vi "Run Tests.vi"(8 "error in (no error)":errorcluster, 10 "Filter":T1, 11 "Execution UI in":refnum<class "Execution UI.lvclass">) -> (0 "error out":errorcluster, 3 "Execution UI out":refnum<class "Execution UI.lvclass">)   [LabVIEW 2020, in "Execution UI.lvclass"]
uses:
  Execution UI.lvclass
  Execution UI.lvclass/Execution UI.ctl
  Process/Process.lvclass
  Result Model by Reference/Result Model by Reference.lvclass
  C:/git/astemes-lunit/source/User Interface/Process/Process.lvclass
  C:/git/astemes-lunit/source/User Interface/Execution UI/Execution UI.lvclass
  C:/git/astemes-lunit/source/Framework/Result Observer/Result Observer.lvclass
  Result Model/Tree Item Filter.ctl
  Result Model/Result Model.lvclass
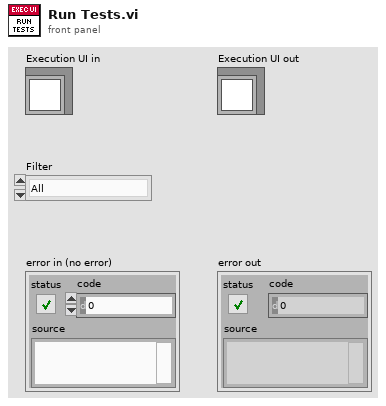
[diagram p1: front panel]
types:
  T1 = typedef "Result Model.lvclass/Tree Item Filter.ctl" = enum16{"All", "Only Fails", "Fails and Not Executed"}
  T2 = cluster{"Left Cell String":string, "Child Text":string[], "Child Tag":string, "Item Indent":i32, "Child Only?":bool, "Glyph Index":i32}[]
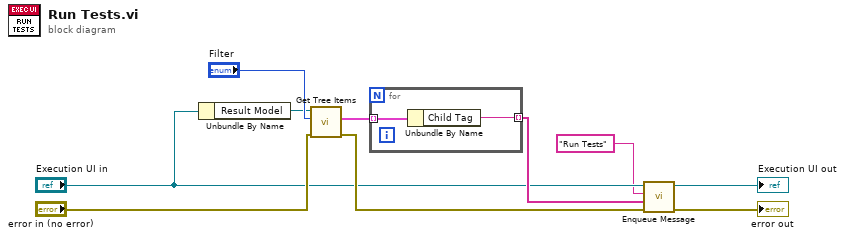
[diagram p0: block diagram]
diagram:
  n1 = Unbundle By Name("Execution UI in") -> ("Result Model"=w5:refnum<class "Result Model by Reference.lvclass">)
  n2 = call "Get Tree Items.vi"("error in (no error)"="error in (no error)", "Filter"="Filter", "Result Model by Reference In"=w5) -> ("error out"=w6:errorcluster, "Tree Items"=w9:T2)  [unwired: 7 in]
  n3 = for {
    tunnel: w9 -> [w12] mode=indexing
    tunnel: [w11] -> w10 mode=indexing
    n4 = Unbundle By Name(w12) -> ("Child Tag"=w11:string)
  }
  n5 = call "Enqueue Message.vi"("error in (no error)"=w6, "Message Data"=w10, "Message"="Run Tests", "Process In"="Execution UI in") -> ("error out"=→"error out":errorcluster, "Process Out"=→"Execution UI out":refnum<class "Execution UI.lvclass">)  [unwired: 6 in]
